vi "Format Tree.vi"(9 "Update":bool, 10 "Commands":T1, 11 "Tree Refnum":refnum<vi>) -> ()   [LabVIEW 2025]
uses:
  Types/Full Command Info.ctl
  Types/Single Cmd Info.ctl
  <vilib>/picture/picture.llb/imagedata.ctl
  de0d8f5a-d376-4f04-a7f2-58c253a07d42.vi
  <vilib>/Utility/Data Type/NI_Data Type.lvlib
panel:
  in  "Tree":string(tree)
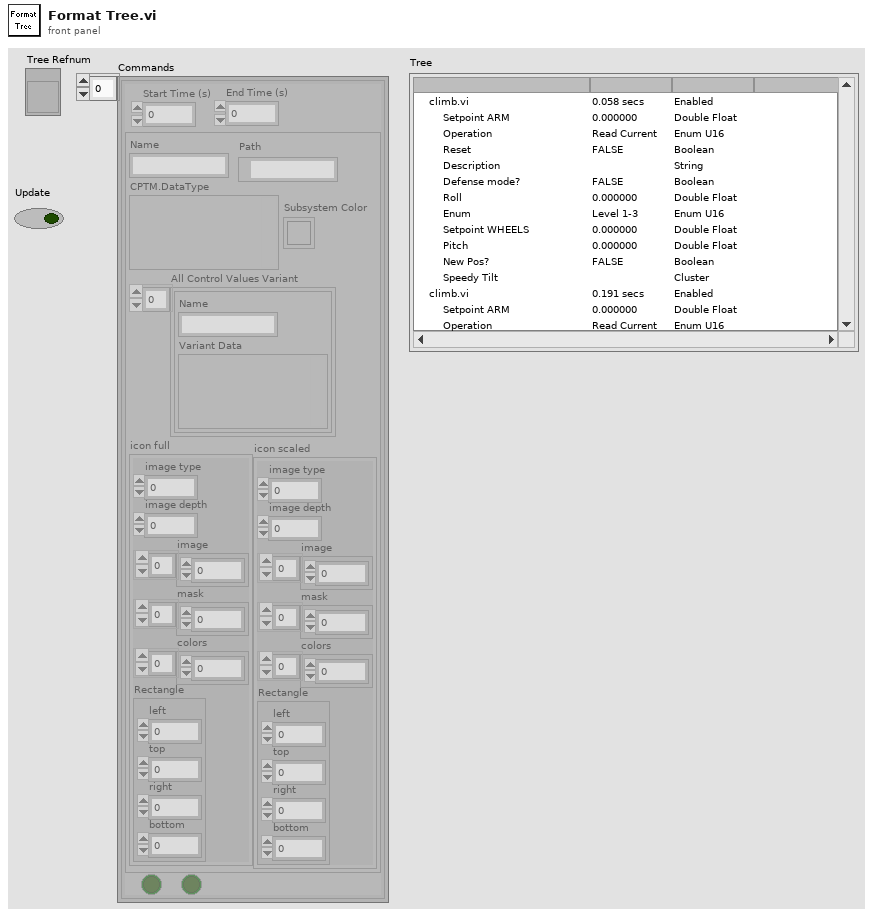
[diagram p1: front panel]
types:
  T1 = typedef "Full Command Info.ctl" = cluster{"Start Time (s)":dbl, "End Time (s)":dbl, T2, "Visible":bool, "Enabled?":bool}[]
  T2 = typedef "Single Cmd Info.ctl" = cluster{"Name":string, "CPTM.DataType":variant, "All Control Values Variant":cluster{"Name":string, "Variant Data":variant}[], "icon full":T3, "icon scaled":T3, "Path":path, "Subsystem Color":u32}
  T3 = typedef "imagedata.ctl" = cluster{"image type":i32, "image depth":i32, "image":u8[], "mask":u8[], "colors":u32[], "Rectangle":cluster{"left":i16, "top":i16, "right":i16, "bottom":i16}}
  T4 = cluster{"Left Cell String":string, "Child Text":string[], "Child Tag":string, "Item Indent":i32, "Child Only?":bool, "Glyph Index":i32}
  T5 = cluster{"Left Cell String":string, "Child Text":string[], "Child Tag":string, "Item Indent":i32, "Child Only?":bool, "Glyph Index":i32}[]
  T6 = typedef "NI_Data Type.lvlib/Data Type.ctl" = enum8{"Invalid Type", "Void", "I8", "I16", "I32", "I64", "U8", "U16", "U32", "U64", "Single Float", "Double Float", "Extended Float", "Single Complex", "Double Complex", "Extended Complex", "Enum U8", "Enum U16", "Enum U32", "Enum U64", "Single Float With Unit", "Double Float With Unit", "Extended Float With Unit", "Single Complex with Unit", "Double Complex with Unit", "Extended Complex with Unit", "Boolean", "String", "Path", "Picture", "Tag", "Array", "Cluster", "Variant", "LV Variant", "Waveform", "Timestamp", "Digital Waveform", "Digital Data", "ExpressData", "Refnum", "External Data", "VI", "Poly VI", "LabVIEW Class Instance", "Fixed Point", "Set Collection", "Map Collection"}
  T7 = typedef "NI_Data Type.lvlib/Type Definition Info.ctl" = cluster{"Name":string, "Timestamp":u32}
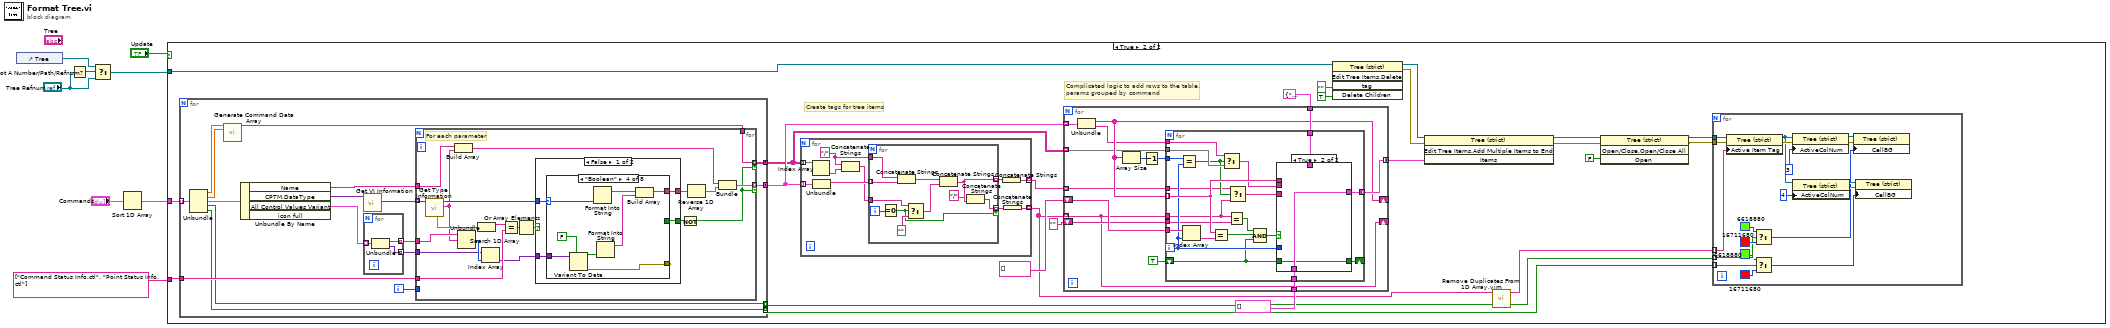
[diagram p0: block diagram]
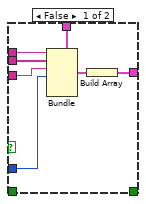
[diagram p3: hidden frame]
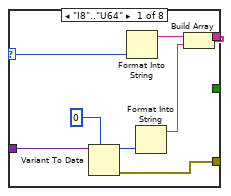
[diagram p4: hidden frame]
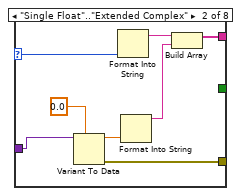
[diagram p5: hidden frame]
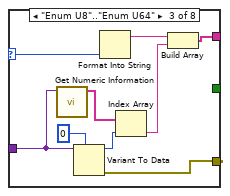
[diagram p6: hidden frame]
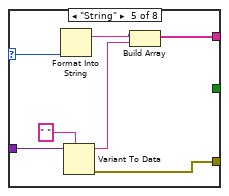
[diagram p7: hidden frame]
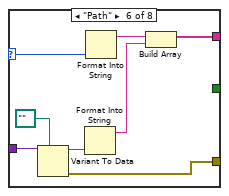
[diagram p8: hidden frame]
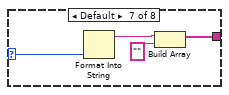
[diagram p9: hidden frame]
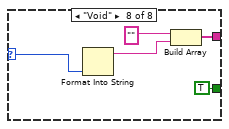
[diagram p10: hidden frame]
diagram:
  n1 = control-ref of="Tree"() -> (w6:refnum<vi>)
  n2 = Not A Number/Path/Refnum?(number/path/refnum="Tree Refnum") -> (NaN/Path/Refnum?=w8:bool)
  n3 = Select(t=w6, s=w8, f="Tree Refnum") -> (s? t:f=w3:refnum<vi>)
  n4 = Sort 1D Array(array="Commands") -> (sorted array=w2:T1)
  n5 = case shown="True" "Update" {
    tunnel: string[] ["Command Status Info.ctl", "Point Status Info.ctl"] ("Name") -> [_ w32]
    tunnel: w3 -> [_ w19]
    tunnel: w2 -> [_ w18]
    frame False {
    }
    frame True {
      # "Complicated logic to add rows to the table,\nparams grouped by command"
      # "Create tags for tree items"
      n6 = for {
        tunnel: [w110] -> w17 mode=concatenating
        tunnel: w32 -> [w105]
        tunnel: w18 -> [w104] mode=indexing
        tunnel: [w101] -> w16 mode=concatenating
        tunnel: [w96] -> w11 mode=indexing
        tunnel: [w97] -> w12 mode=indexing
        i -> [w106]
        n7 = Unbundle(w104) -> ("Start Time (s)"=w100:dbl, "End Time (s)"=w99:dbl, w98:T2, "Visible"=w97:bool, "Enabled?"=w96:bool)
        n8 = call "Generate Command Data Array.vi"("Start Time (s)"=w100, "End Time (s)"=w99) -> ("Array"=w102:string[])  [unwired: 13 in]
        n9 = Unbundle By Name(w98) -> ("Name"=w103:string, "CPTM.DataType"=w112:variant, "All Control Values Variant"=w109:cluster{"Name":string, "Variant Data":variant}[])  [unwired: 1 out]
        n10 = call <vilib>:"Get VI Information.vi"("variant"=w112) -> ("VI terminal types"=w111:variant[])  [unwired: 7 in, 3 out]
        n11 = for {
          tunnel: w109 -> [w197] mode=indexing
          tunnel: [w196] -> w108 mode=indexing
          tunnel: [w195] -> w107 mode=indexing
          n12 = Unbundle(w197) -> ("Name"=w196:string, "Variant Data"=w195:variant)
        }
        n13 = for {
          tunnel: w111 -> [w132] mode=indexing
          tunnel: [w129] -> w110 mode=indexing if=w115
          tunnel: w105 -> [w127]
          tunnel: w108 -> [w123]
          tunnel: w107 -> [w120]
          tunnel: w106 -> [_]
          tunnel: w103 -> [w118]
          tunnel: w102 -> [w116]
          tunnel: [w116] -> w101 mode=indexing if=w115
          # "For each parameter"
          n14 = call <vilib>:"Get Type Information.vi"("variant"=w132) -> ("name"=w122:string, "type"=w131:T6, "type definition info"=w128:T7)  [unwired: 6 in, 2 out]
          n15 = Build Array(w118, w122) -> (w130:string[])
          n16 = Search 1D Array(1D array=w123, element=w122) -> (index of element=w121:i32)  [unwired: 1 in]
          n17 = Unbundle(w128) -> ("Name"=w126:string)  [unwired: 1 out]
          n18 = Index Array(array=w120, index=w121) -> (element=w119:variant)
          n19 = Equal?(x=w126, y=w127) -> (x = y?=w114:bool[])
          n20 = Or Array Elements(Boolean array=w114) -> (logical OR=w113:bool)
          n21 = case shown="False" w113 {
            selector: w113 -> [_ w194]
            tunnel: w131 -> [w136 _]
            tunnel: [w135 _] -> w124
            tunnel: [w134 w194] -> w125
            tunnel: w119 -> [w133 _]
            frame False {
              n22 = case shown="\"Boolean\"" w136 {
                selector: w136 -> [w144 w152 w161 w169 w176 w184 w188 w193]
                tunnel: [w139 w146 w158 w164 w173 w179 w186 w190] -> w135
                tunnel: [_ _ _ _ _ _ _ TRUE] -> w134
                tunnel: w133 -> [w138 w149 w156 w166 w175 w181 _ _]
                tunnel: [w137 w145 w157 w162 w170 w177 _ _] -> _
                frame "I8".."U64" {
                  n23 = Variant To Data(type=i64 0, Variant=w138) -> (data=w142:i64, error out=w137:errorcluster)  [unwired: 1 in]
                  n24 = Format Into String(w144) -> (resulting string=w140:string)  [unwired: 3 in, 1 out]
                  n25 = Format Into String(w142) -> (resulting string=w141:string)  [unwired: 3 in, 1 out]
                  n26 = Build Array(w140, w141) -> (w139:string[])
                }
                frame "Single Float".."Extended Complex" {
                  n27 = Variant To Data(type=0.0, Variant=w149) -> (data=w150:dbl, error out=w145:errorcluster)  [unwired: 1 in]
                  n28 = Format Into String(w152) -> (resulting string=w148:string)  [unwired: 3 in, 1 out]
                  n29 = Format Into String(w150) -> (resulting string=w147:string)  [unwired: 3 in, 1 out]
                  n30 = Build Array(w148, w147) -> (w146:string[])
                }
                frame "Enum U8".."Enum U64" {
                  n31 = call <vilib>:"Get Numeric Information.vi"("variant"=w156) -> ("enum names"=w155:string[])  [unwired: 7 in, 3 out]
                  n32 = Variant To Data(type=i64 0, Variant=w156) -> (data=w154:i64, error out=w157:errorcluster)  [unwired: 1 in]
                  n33 = Format Into String(w161) -> (resulting string=w159:string)  [unwired: 3 in, 1 out]
                  n34 = Index Array(array=w155, index=w154) -> (element=w153:string)
                  n35 = Build Array(w159, w153) -> (w158:string[])
                }
                frame "Boolean" {
                  n36 = Variant To Data(type=FALSE, Variant=w166) -> (data=w167:bool, error out=w162:errorcluster)  [unwired: 1 in]
                  n37 = Format Into String(w169) -> (resulting string=w165:string)  [unwired: 3 in, 1 out]
                  n38 = Format Into String(w167) -> (resulting string=w163:string)  [unwired: 3 in, 1 out]
                  n39 = Build Array(w165, w163) -> (w164:string[])
                }
                frame "String" {
                  n40 = Format Into String(w176) -> (resulting string=w174:string)  [unwired: 3 in, 1 out]
                  n41 = Variant To Data(type=" ", Variant=w175) -> (data=w172:string, error out=w170:errorcluster)  [unwired: 1 in]
                  n42 = Build Array(w174, w172) -> (w173:string[])
                }
                frame "Path" {
                  n43 = Variant To Data(type=path "", Variant=w181) -> (data=w182:path, error out=w177:errorcluster)  [unwired: 1 in]
                  n44 = Format Into String(w182) -> (resulting string=w178:string)  [unwired: 3 in, 1 out]
                  n45 = Format Into String(w184) -> (resulting string=w180:string)  [unwired: 3 in, 1 out]
                  n46 = Build Array(w180, w178) -> (w179:string[])
                }
                frame Default {
                  n47 = Format Into String(w188) -> (resulting string=w187:string)  [unwired: 3 in, 1 out]
                  n48 = Build Array(w187, "") -> (w186:string[])
                }
                frame "Void" {
                  n49 = Format Into String(w193) -> (resulting string=w191:string)  [unwired: 3 in, 1 out]
                  n50 = Build Array("", w191) -> (w190:string[])
                }
              }
            }
            frame True {
            }
          }
          n51 = Not(x=w125) -> (.not. x?=w115:bool)
          n52 = Reverse 1D Array(array=w124) -> (reversed array=w117:string[])
          n53 = Bundle(w130, w117) -> (w129:cluster{string[], string[]})  [unwired: 1 in]
        }
      }
      n54 = for {
        tunnel: w17 -> [w207] mode=indexing
        tunnel: [w204] -> w29 mode=indexing
        tunnel: w16 -> [w203] mode=indexing
        tunnel: [w199] -> w14 mode=indexing
        w198 = "/"
        n55 = Index Array(array=w203) -> (element=w202:string)  [unwired: 1 in]
        n56 = Unbundle(w207) -> (w206:string[])  [unwired: 1 out]
        n57 = Concatenate Strings(w198, w202) -> (w201:string)
        n58 = for {
          tunnel: w206 -> [w218] mode=indexing
          tunnel: [w211] -> w205 mode=indexing
          tunnel: w201 -> [w214]
          tunnel: [w210] -> w200 mode=indexing if=w212
          tunnel: w198 -> [w208]
          i -> [w217]
          n59 = Equal To 0?(x=w217) -> (x = 0?=w212:bool)
          n60 = Concatenate Strings(w208, w218) -> (w216:string)
          n61 = Select(t=w214, s=w212, f="") -> (s? t:f=w213:string)
          n62 = Concatenate Strings(w216, w213) -> (w211:string)
          n63 = Concatenate Strings("/", w211) -> (w210:string)
        }
        n64 = Concatenate Strings(w205) -> (w204:string)
        n65 = Concatenate Strings(w200) -> (w199:string)
      }
      n66 = for {
        tunnel: [w61] -> w20 mode=concatenating
        tunnel: T4 {"Left Cell String"="", "Child Text"=[], "Child Tag"="", "Item Indent"=0, "Child Only?"=FALSE, "Glyph Index"=0} ("Item") -> [w62]
        shift-right: [w58] -> _
        shift-left: string[] [] ("Child Text") -> [w64]
        tunnel: w17 -> [w65] mode=indexing
        tunnel: T5 [] -> [w63]
        tunnel: w29 -> [w57] mode=indexing
        tunnel: w16 -> [w54] mode=indexing
        tunnel: w14 -> [w52] mode=indexing
        shift-right: [w52] -> _
        shift-left: "" -> [w53]
        n67 = Unbundle(w65) -> (w58:string[], w55:string[])
        n68 = Array Size(array=w58) -> (size(s)=w60:i32)
        n69 = Decrement(x=w60) -> (x-1=w59:i32)
        n70 = for {
          tunnel: w64 -> [w86]
          tunnel: w58 -> [w81] mode=indexing
          tunnel: w63 -> [w84]
          tunnel: [w83] -> w61 mode=concatenating
          tunnel: w62 -> [w82]
          tunnel: w59 -> [w79]
          tunnel: w55 -> [w73]
          tunnel: w57 -> [w69]
          shift-right: [w76] -> _
          shift-left: TRUE -> [w75]
          tunnel: w54 -> [w72]
          tunnel: w52 -> [w68]
          tunnel: w53 -> [w67]
          i -> [w80]
          n71 = Equal?(x=w79, y=w80) -> (x = y?=w71:bool)
          n72 = Index Array(array=w86, index=w80) -> (element=w85:string)
          n73 = Equal?(x=w81, y=w85) -> (x = y?=w78:bool)
          n74 = Select(t=w73, s=w71, f=w72) -> (s? t:f=w74:string[])
          n75 = Equal?(x=w68, y=w67) -> (x = y?=w66:bool)
          n76 = Select(t=w69, s=w71, f=w68) -> (s? t:f=w70:string)
          n77 = Compound Arithmetic op=AND(w66, w78, w75) -> (w77:bool)
          n78 = case shown="True" w77 {
            tunnel: [w91 w95] -> w83
            tunnel: w84 -> [_ w95]
            tunnel: w82 -> [w93 _]
            tunnel: w81 -> [w90 _]
            tunnel: w80 -> [w89 _]
            tunnel: w74 -> [w88 _]
            tunnel: w70 -> [w87 _]
            tunnel: [_ w94] -> w76
            tunnel: w75 -> [_ w94]
            frame False {
              n79 = Bundle(cluster=w93, "Left Cell String"=w90, "Child Text"=w88, "Child Tag"=w87, "Item Indent"=w89) -> (w92:T4)  [unwired: 2 in]
              n80 = Build Array(w92) -> (w91:T5)
            }
            frame True {
            }
          }
        }
      }
      n81 = invoke on="Invoke Node" class="Tree (strict)" method="Edit Tree Items.Delete"(reference=w19, "tag"="" ("Tag"), "Delete Children"=TRUE ("Delete Children?")) -> (reference out=w26:refnum<vi>, error out=w21:errorcluster)  [unwired: 2 in, 3 out]
      n82 = invoke on="Invoke Node" class="Tree (strict)" method="Edit Tree Items.Add Multiple Items to End"(reference=w26, error in=w21, "Items"=w20) -> (reference out=w27:refnum<vi>, error out=w24:errorcluster)  [unwired: 1 in, 2 out]
      n83 = call "Remove Duplicates From 1D Array.vim"("array"=w14) -> ("array with duplicates removed"=w13:string[])  [unwired: 10 in]
      n84 = invoke on="Invoke Node" class="Tree (strict)" method="Open/Close.Open/Close All"(reference=w27, error in=w24, "Open"=FALSE ("Open?")) -> (reference out=w10:refnum<vi>, error out=w9:errorcluster)  [unwired: 1 in, 2 out]
      n85 = for {
        tunnel: w13 -> [w50] mode=indexing
        tunnel: w12 -> [w45] mode=indexing
        tunnel: w11 -> [w42] mode=indexing
        tunnel: w10 -> [w51]
        tunnel: w9 -> [w48]
        n86 = property class="Tree (strict)"(reference=w51, error in=w48, "Active Item Tag"=w50) -> (reference out=w36:refnum<vi>, error out=w49:errorcluster)
        n87 = Select(t=u32 6618880, s=w45, f=u32 16711680) -> (s? t:f=w34:u32)
        n88 = Select(t=u32 6618880, s=w42, f=u32 16711680) -> (s? t:f=w33:u32)
        n89 = property class="Tree (strict)"(reference=w36, error in=w49, "ActiveColNum"=3 ("Active Cell:Active Column Number")) -> (reference out=w41:refnum<vi>, error out=w40:errorcluster)
        n90 = property class="Tree (strict)"(reference=w36, "ActiveColNum"=4 ("Active Cell:Active Column Number")) -> (reference out=w38:refnum<vi>, error out=w37:errorcluster)  [unwired: 1 in]
        n91 = property class="Tree (strict)"(reference=w41, error in=w40, "CellBG"=w34) -> ()  [unwired: 2 out]
        n92 = property class="Tree (strict)"(reference=w38, error in=w37, "CellBG"=w33) -> ()  [unwired: 2 out]
      }
    }
  }
